vi "CB Local Sense Test.vi"(5 "HMP4040 Channel Settings":T2={"CH1 Voltage"=24.0, "CH1 Current"=1.0, "CH1 Output"=TRUE, "CH2 Voltage"=24.0, "CH2 Current"=1.0, "CH2 Output"=TRUE, "CH3 Voltage"=24.0, "CH3 Current"=1.0, "CH3 Output"=TRUE, "CH4 Voltage"=24.0, "CH4 Current"=1.0, "CH4 Output"=TRUE, "Master Output"=TRUE} {"CH4 Current" format="%.3f"; "CH4 Voltage" format="%.3f"; "CH3 Current" format="%.3f"; "CH3 Voltage" format="%.3f"; "CH2 Current" format="%.3f"; "CH2 Voltage" format="%.3f"; "CH1 Current" format="%.3f"; "CH1 Voltage" format="%.3f"}, 8 "error in (no error)":errorcluster, 9 "Board Selector":T1, 10 "Message IN":string) -> (0 "error out":errorcluster, 1 "Pass?":bool, 2 "Message OUT":string)   [LabVIEW 2022 SP3]
uses:
  HMP4000 Communication/HMP4040_ChannelControl.ctl
  Serial Board Com/Board Select.ctl
panel:
  out "MSE Array":dbl[](array[numeric])
  out "Voltage Readings":dbl[][](array[numeric])
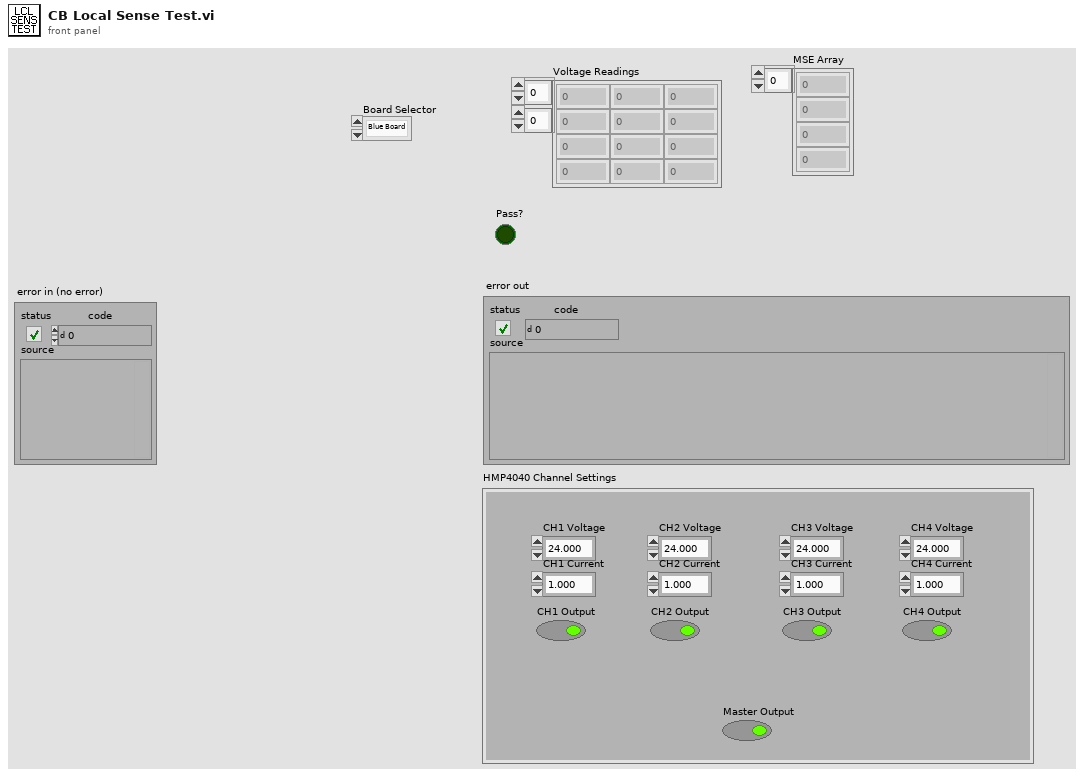
[diagram p1: front panel]
types:
  T1 = typedef "Board Select.ctl" = enum16{"Blue Board", "Green Board"}
  T2 = typedef "HMP4040_ChannelControl.ctl" = cluster{"CH1 Voltage":dbl, "CH1 Current":dbl, "CH1 Output":bool, "CH2 Voltage":dbl, "CH2 Current":dbl, "CH2 Output":bool, "CH3 Voltage":dbl, "CH3 Current":dbl, "CH3 Output":bool, "CH4 Voltage":dbl, "CH4 Current":dbl, "CH4 Output":bool, "Master Output":bool}
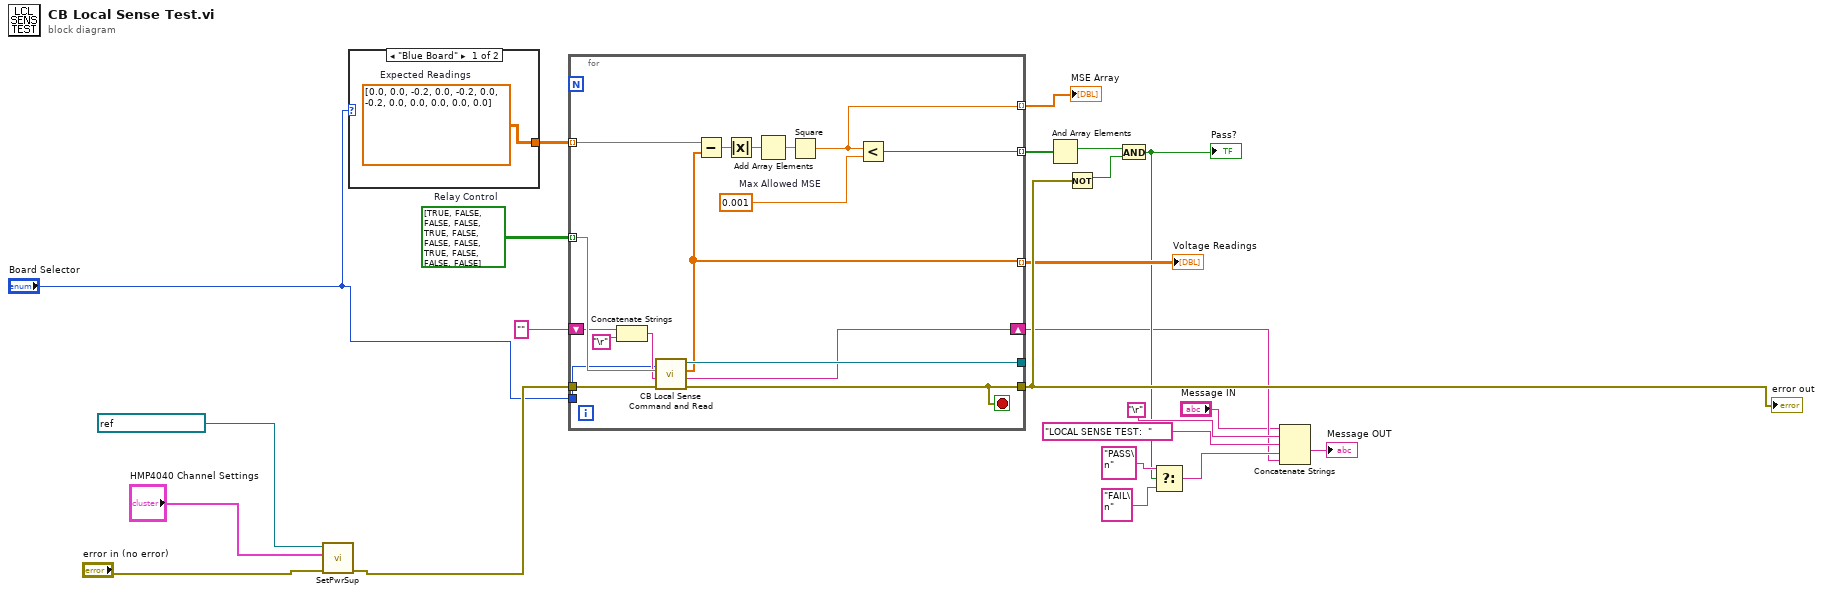
[diagram p0: block diagram]
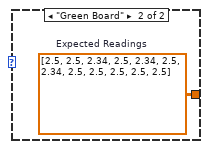
[diagram p2: hidden frame]
diagram:
  w21 = bool[][] [[TRUE, FALSE, FALSE], [FALSE, TRUE, FALSE], [FALSE, FALSE, TRUE], [FALSE, FALSE, FALSE]]  # Relay Control
  n1 = call "SetPwrSup.vi"("error in (no error)"="error in (no error)", "HMP4040 Channel Settings"="HMP4040 Channel Settings", "HMP4040 IN"=refnum<visa-resource-name> "HMP4040_FTS2" ("VISA resource name")) -> ("error out"=w4:errorcluster)  [unwired: 7 in, 1 out]
  n2 = case shown="\"Blue Board\"" "Board Selector" {
    tunnel: [w24 w25] -> w23
    frame "Blue Board" {
      w24 = dbl[][] [[0.0, 0.0, -0.2], [0.0, -0.2, 0.0], [-0.2, 0.0, 0.0], [0.0, 0.0, 0.0]]  # Expected Readings
    }
    frame "Green Board" {
      w25 = dbl[][] [[2.5, 2.5, 2.34], [2.5, 2.34, 2.5], [2.34, 2.5, 2.5], [2.5, 2.5, 2.5]]  # Expected Readings
    }
  }
  n3 = for {
    tunnel: [w40] -> w18
    tunnel: [w42] -> _
    tunnel: w4 -> [w41]
    tunnel: w23 -> [w37] mode=indexing
    tunnel: [w34] -> w22 mode=indexing
    tunnel: w21 -> [w33] mode=indexing
    tunnel: [w32] -> w17 mode=indexing
    tunnel: [w31] -> w16 mode=indexing
    shift-right: [w30] -> w9
    shift-left: "" -> [w29]
    tunnel: "Board Selector" -> [w26]
    stop <- w40 stop-if-true
    w35 = 0.001  # Max Allowed MSE
    n4 = Concatenate Strings(w29, "\r") -> (w28:string)
    n5 = call "CB Local Sense Command and Read.vi"("Board Selector"=w26, "error in (no error)"=w41, "Message IN"=w28, "Relay Control"=w33) -> ("error out"=w40:errorcluster, "Message OUT"=w30:string, "Voltage Array"=w32:dbl[], "Control Board OUT"=w42:refnum<visa-resource-name>)  [unwired: 4 in]
    n6 = Subtract(x=w37, y=w32) -> (x-y=w39:dbl[])
    n7 = Absolute Value(x=w39) -> (abs(x)=w38:dbl[])
    n8 = Add Array Elements(numeric array=w38) -> (sum=w36:dbl)
    n9 = Square(x=w36) -> (x^2=w31:dbl)
    n10 = Less?(x=w31, y=w35) -> (x < y?=w34:bool)
  }
  "error out" <- w18
  "Voltage Readings" <- w17
  "MSE Array" <- w16
  n11 = And Array Elements(Boolean array=w22) -> (logical AND=w20:bool)
  n12 = Not(x=w18) -> (.not. x?=w19:bool)
  n13 = And(x=w20, y=w19) -> (x .and. y?=w11:bool)
  "Pass?" <- w11
  n14 = Select(t="PASS\n", s=w11, f="FAIL\n") -> (s? t:f=w10:string)
  n15 = Concatenate Strings("Message IN", "\r", "LOCAL SENSE TEST:  ", w10, w9) -> (→"Message OUT":string)
